vi "Example 1.vi"(8 "error in (no error)":errorcluster) -> (0 "error out":errorcluster)   [LabVIEW 2021, in "Named Counters.lvlib"]
uses:
  Named Counters.lvlib
panel:
  out "Number of counters":i32
  out "counters":string[](array[string])
  in  "Use case":enum16{"Use case 1", "Use case 2", "Use case 3"}(ring)
  out "Counter 3":i32
  out "Counter 2":i32
  out "Counter 1":i32
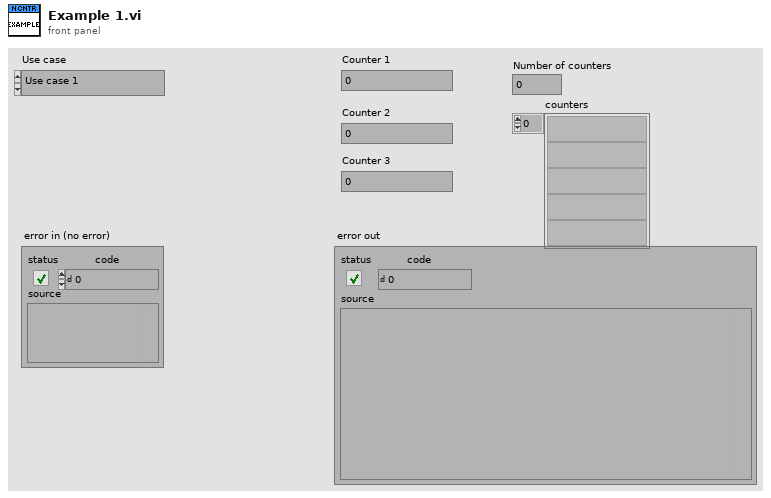
[diagram p1: front panel]
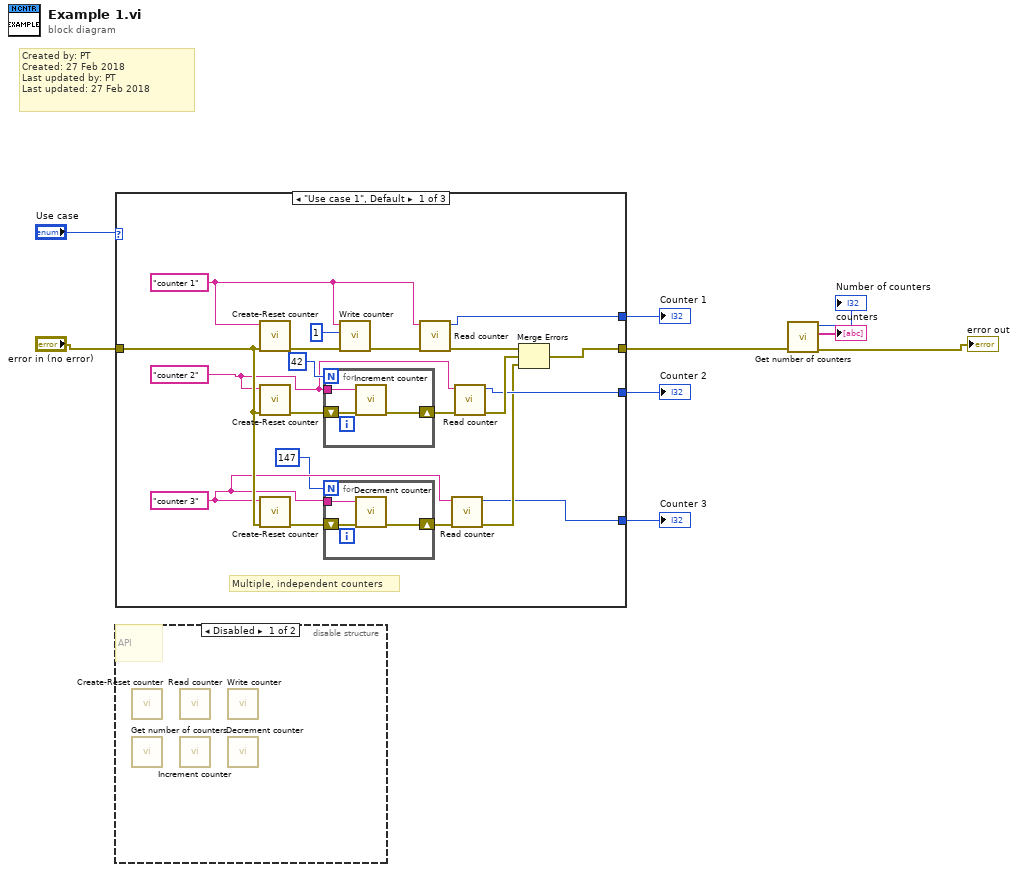
[diagram p0: block diagram]
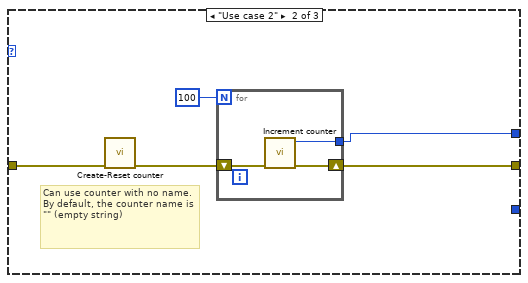
[diagram p3: hidden frame]
diagram:
  # "Created by: PT\nCreated: 27 Feb 2018\nLast updated by: PT\nLast updated: 27 Feb 2018"
  n1 = case shown="\"Use case 1\", Default" "Use case" {
    tunnel: [w22 w38 w44] -> w9
    tunnel: "error in (no error)" -> [w29 w40 w44]
    tunnel: [w11 _ _] -> w5
    tunnel: [w17 _ _] -> w4
    tunnel: [w23 w36 _] -> w3
    frame "Use case 1", Default {
      w12 = "counter 3" ("Timer name")
      w16 = "counter 2" ("Timer name")
      w25 = "counter 1" ("Timer name")
      # "Multiple, independent counters"
      n2 = call "Create-Reset counter.vi"("error in (no error)"=w29, "Counter name (dflt=blank)"=w25) -> ("error out"=w28:errorcluster)  [unwired: 9 in]
      n3 = call "Create-Reset counter.vi"("error in (no error)"=w29, "Counter name (dflt=blank)"=w16) -> ("error out"=w21:errorcluster)  [unwired: 9 in]
      n4 = call "Create-Reset counter.vi"("error in (no error)"=w29, "Counter name (dflt=blank)"=w12) -> ("error out"=w15:errorcluster)  [unwired: 9 in]
      n5 = for {
        N: 42 -> [_]
        shift-right: [w33] -> w19
        shift-left: w21 -> [w35]
        tunnel: w16 -> [w34]
        n6 = call "Increment counter.vi"("error in (no error)"=w35, "Counter name (dflt=blank)"=w34) -> ("error out"=w33:errorcluster)  [unwired: 8 in, 1 out]
      }
      n7 = for {
        N: 147 -> [_]
        shift-right: [w30] -> w14
        shift-left: w15 -> [w32]
        tunnel: w12 -> [w31]
        n8 = call "Decrement counter.vi"("error in (no error)"=w32, "Counter name (dflt=blank)"=w31) -> ("error out"=w30:errorcluster)  [unwired: 9 in]
      }
      n9 = call "Write counter.vi"("error in (no error)"=w28, "Value"=1, "Counter name (dflt=blank)"=w25) -> ("error out"=w26:errorcluster)  [unwired: 8 in]
      n10 = call "Read counter.vi"("error in (no error)"=w26, "Counter name (dflt=blank)"=w25) -> ("error out"=w27:errorcluster, "Value"=w23:i32)  [unwired: 8 in]
      n11 = call "Read counter.vi"("error in (no error)"=w14, "Counter name (dflt=blank)"=w12) -> ("error out"=w13:errorcluster, "Value"=w11:i32)  [unwired: 8 in]
      n12 = call "Read counter.vi"("error in (no error)"=w19, "Counter name (dflt=blank)"=w16) -> ("error out"=w18:errorcluster, "Value"=w17:i32)  [unwired: 8 in]
      n13 = Merge Errors(w27, w18, w13) -> (w22:errorcluster)
    }
    frame "Use case 2" {
      # "Can use counter with no name. By default, the counter name is \"\" (empty string)"
      n14 = call "Create-Reset counter.vi"("error in (no error)"=w40) -> ("error out"=w39:errorcluster)  [unwired: 10 in]
      n15 = for {
        N: 100 -> [_]
        shift-right: [w42] -> w38
        shift-left: w39 -> [w43]
        tunnel: [w41] -> w36
        n16 = call "Increment counter.vi"("error in (no error)"=w43) -> ("error out"=w42:errorcluster, "Value (after increment)"=w41:i32)  [unwired: 9 in]
      }
    }
    frame "Use case 3" {
    }
  }
  "Counter 1" <- w3
  "Counter 2" <- w4
  "Counter 3" <- w5
  n17 = disable-structure shown="Disabled" {
    frame Disabled {
      # "API"
      n18 = call "Create-Reset counter.vi"() -> ()  [unwired: 11 in, 1 out]
      n19 = call "Get number of counters.vi"() -> ()  [unwired: 9 in, 3 out]
      n20 = call "Read counter.vi"() -> ()  [unwired: 10 in, 2 out]
      n21 = call "Increment counter.vi"() -> ()  [unwired: 10 in, 2 out]
      n22 = call "Write counter.vi"() -> ()  [unwired: 11 in, 1 out]
      n23 = call "Decrement counter.vi"() -> ()  [unwired: 11 in, 1 out]
    }
    frame Enabled {
    }
  }
  n24 = call "Get number of counters.vi"("error in (no error)"=w9) -> ("error out"=→"error out":errorcluster, "Counters"=→"counters":string[], "Number of counters"=→"Number of counters":i32)  [unwired: 8 in]
